vi "Parse Response JSON.vi"(8 "error in (no error)":errorcluster, 10 "Response JSON":string, 11 "RGetSourceScreenshot in":refnum<class "RGetSourceScreenshot.lvclass">) -> (0 "error out":errorcluster, 3 "RGetSourceScreenshot out":refnum<class "RGetSourceScreenshot.lvclass">)   [LabVIEW 2022 SP3, in "obs-websocket-lv.lvlib" / "RGetSourceScreenshot.lvclass"]
uses:
  RGetSourceScreenshot.lvclass
  RGetSourceScreenshot.lvclass/RGetSourceScreenshot.ctl
  <vilib>/IlluminatedG/lv-web-crypto/lv-json/JSON/JSON.lvlib
  <vilib>/IlluminatedG/lv-web-crypto/lv-base64/Base64.lvlib
  <vilib>/wsapi/NI_WebServices.lvlib
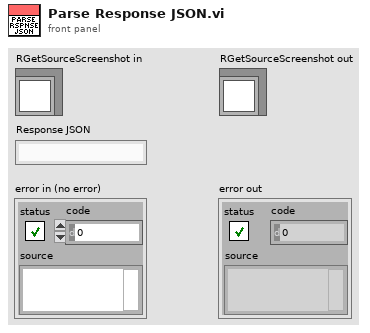
[diagram p1: front panel]
types:
  T1 = typedef "JSON.lvlib/JSON Item Type.ctl" = enum16{"unknown", "null", "Array", "Object", "String", "Number", "Boolean"}
  T2 = typedef "imagedata.ctl" = cluster{"image type":i32, "image depth":i32, "image":u8[], "mask":u8[], "colors":u32[], "Rectangle":cluster{"left":i16, "top":i16, "right":i16, "bottom":i16}}
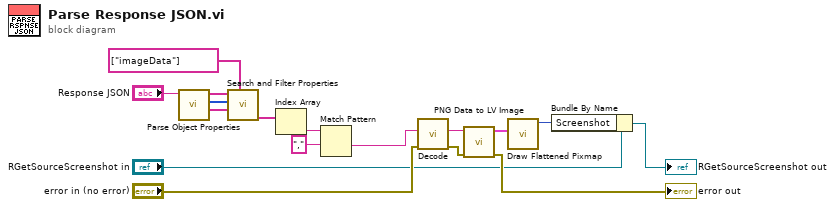
[diagram p0: block diagram]
diagram:
  n1 = call <vilib>:"Parse Object Properties.vi"("JSON String"="Response JSON") -> ("Values"=w11:string[], "Item Types"=w12:T1[], "Keys"=w13:string[])  [unwired: 7 in, 1 out]
  n2 = call <vilib>:"Search and Filter Properties.vi"("Search Keys"=string[] ["imageData"], "Values In"=w11, "Types In"=w12, "Keys In"=w13) -> ("Filtered Values"=w9:string[])  [unwired: 2 in, 5 out]
  n3 = Index Array(array=w9) -> (element=w3:string)  [unwired: 1 in]
  n4 = Match Pattern(string=w3, regular expression=",") -> (after substring=w1:string)  [unwired: 1 in, 3 out]
  n5 = call <vilib>:"Decode.vi"("error in (no error)"="error in (no error)", "string in (base64-encoded)"=w1) -> ("error out"=w4:errorcluster, "string out (decoded)"=w8:string)  [unwired: 8 in]
  n6 = call <vilib>:"PNG Data to LV Image.vi"("error in (no error)"=w4, "png data"=w8) -> ("error out"=→"error out":errorcluster, "image data"=w7:T2)  [unwired: 8 in]
  n7 = call <vilib>:"Draw Flattened Pixmap.vi"("image data"=w7) -> ("new picture"=w5:picture)  [unwired: 8 in]
  n8 = Bundle By Name(cluster="RGetSourceScreenshot in", "Screenshot"=w5) -> (→"RGetSourceScreenshot out":refnum<class "RGetSourceScreenshot.lvclass">)
